vi "AssertsVIExecStateIdle.vi"(0 "VI Reference In":refnum<vi>, 1 "Label (VI Title)":string="Default", 11 "error in":errorcluster) -> (4 "VI Reference Out":refnum<vi>, 15 "error out":errorcluster)   [LabVIEW 2016, in "DronaTest.lvlib"]
uses:
  DronaTest.lvlib
  APIs/Stimulus/ControlValue/ValueSignalLatchBooleanString.vi
  <vilib>/addons/_JKI Toolkits/Caraya/classes/Assert/Assert Not Error.vi
  APIs/Assert/AssertVI/AssertVIExecIdle.vi
  <vilib>/addons/_JKI Toolkits/Caraya/classes/Test/Test.lvclass
  Drona.lvlib
  <vilib>/addons/_JKI Toolkits/Caraya/classes/Assert/Assert.lvclass
  APIs/Stimulus/ControlValue/ControlValue.lvlib
  APIs/Assert/AssertVI/AssertVI.lvlib
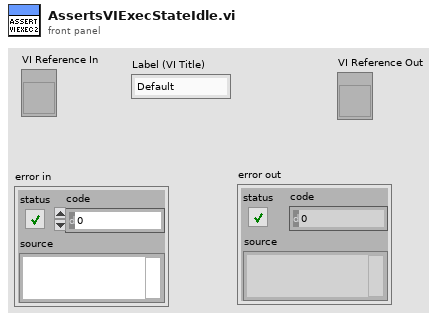
[diagram p1: front panel]
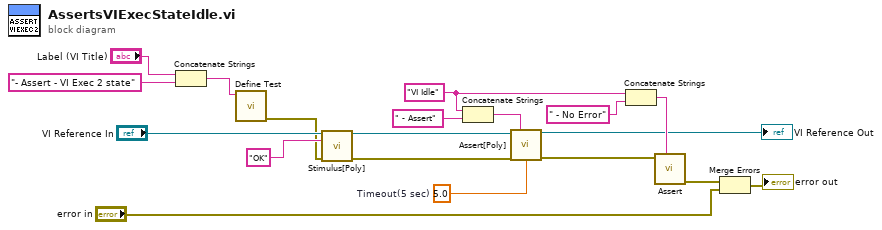
[diagram p0: block diagram]
diagram:
  w13 = "VI Idle" ("Label")
  w10 = 5.0  # Timeout(5 sec)
  n1 = Concatenate Strings("Label (VI Title)", "- Assert - VI Exec 2 state" ("string")) -> (w16:string)
  n2 = call <vilib>:"Define Test.vi"("Label (VI Title)"=w16) -> ("error out"=w2:errorcluster)  [unwired: 10 in]
  n3 = call-poly "Stimulus[Poly].vi"("VI Reference In"="VI Reference In", "Control Path"="OK", "error in"=w2) -> ("VI Reference Out"=w5:refnum<vi>, "error out"=w7:errorcluster)  [unwired: 11 in]
  n4 = Concatenate Strings(w13, " - Assert" ("string")) -> (w11:string)
  n5 = call-poly "Assert[Poly].vi"("VI Reference In"=w5, "Test Label"=w11, "Error In"=w7, "Timeout(5 sec)"=w10) -> ("VI Reference Out"=→"VI Reference Out":refnum<vi>, "Error Out"=w8:errorcluster)  [unwired: 10 in]
  n6 = Concatenate Strings(w13, " - No Error" ("string")) -> (w19:string)
  n7 = call-poly <vilib>:"Assert.vi"("Label"=w19, "Not Error?"=w8) -> ("error out"=w4:errorcluster)  [unwired: 9 in]
  n8 = Merge Errors(w4, "error in") -> (→"error out":errorcluster)
